vi "Facade.vi"(0 "Data In":T4, 2 "Display State In":T2, 3 "Container State":T3) -> (6 "Data Out":T4, 7 "Display State Out":T2, 8 "Action":T1)   [LabVIEW 2015, in "Scale Selector.xctl"]
uses:
  Scale Selector.xctl
  Data.vi
  <vilib>/_xctls/Container State.ctl
  State.vi
  <vilib>/_xctls/Action.ctl
  <vilib>/_xctls/XControlSupport.lvlib
panel:
  in  "Down Button":bool
  in  "Up Button":bool
  in  "Scale":dbl format="%#pV"
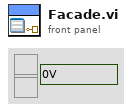
[diagram p1: front panel]
types:
  T1 = typedef "XControlSupport.lvlib/Action.ctl" = cluster{"Data Changed?":bool, "State Changed?":bool, "Action Name":string}
  T2 = typedef "Scale Selector.xctl/State.vi" = cluster{"scale":enum16{"Linear", "Log"}, "increment":dbl}
  T3 = typedef "XControlSupport.lvlib/Container State.ctl" = cluster{"Indicator?":bool, "Run Mode?":bool, " Refnum":refnum<vi>}
  T4 = typedef "Scale Selector.xctl/Data.vi" = dbl
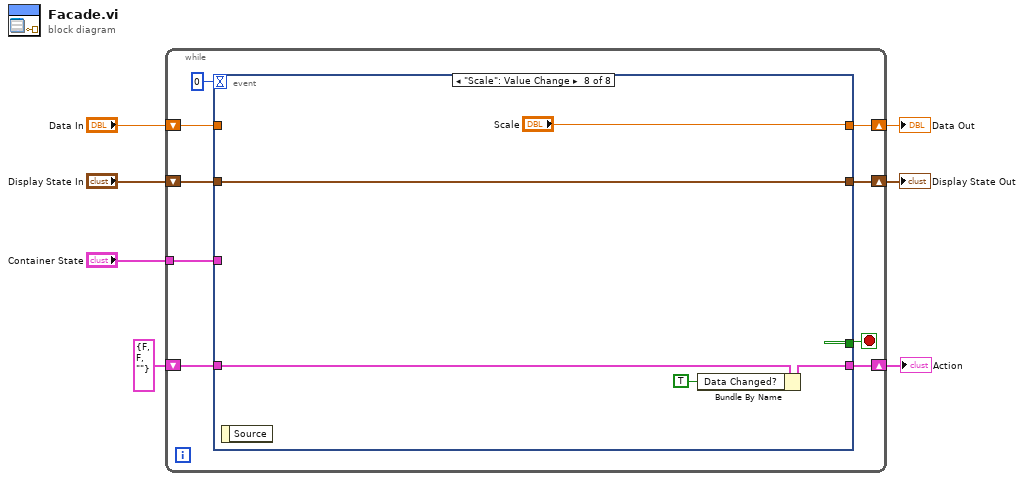
[diagram p0: block diagram]
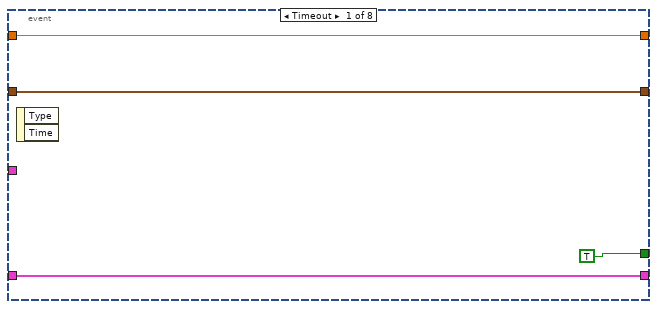
[diagram p2: hidden frame]
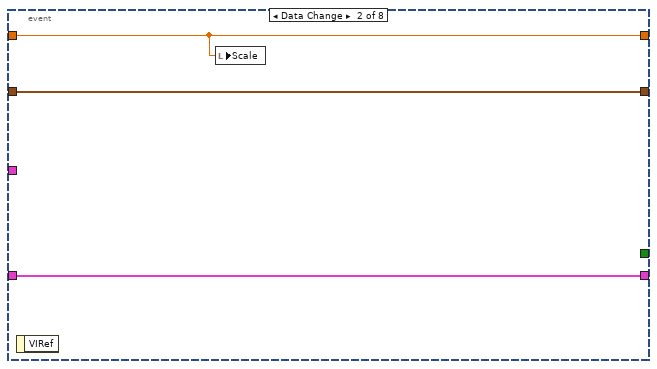
[diagram p3: hidden frame]
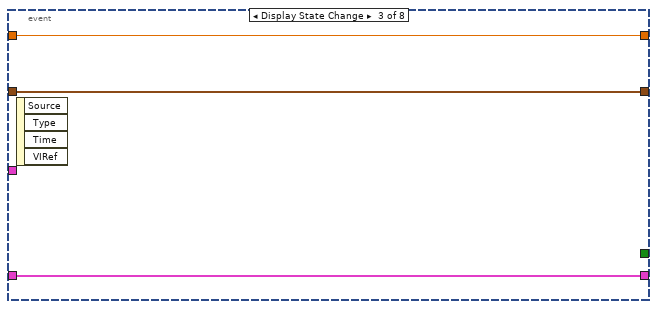
[diagram p4: hidden frame]
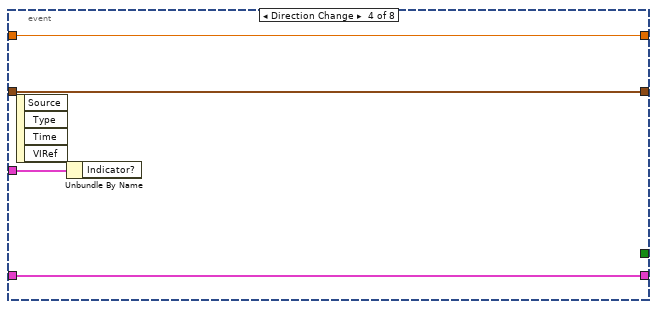
[diagram p5: hidden frame]
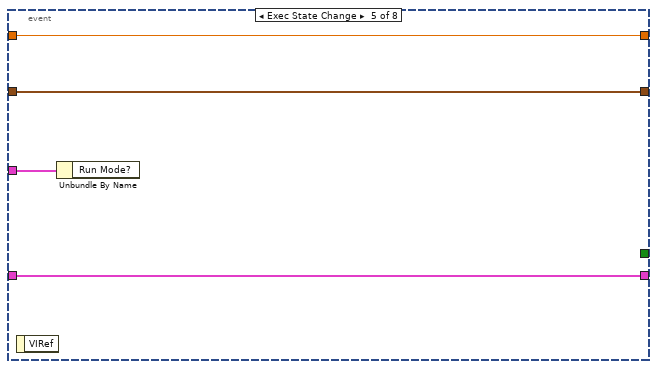
[diagram p6: hidden frame]
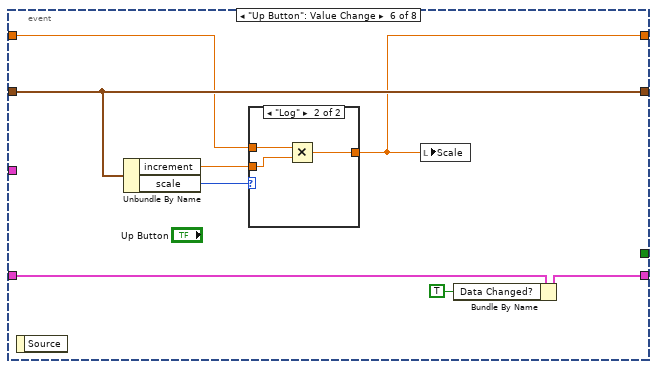
[diagram p7: hidden frame]
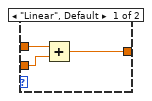
[diagram p8: hidden frame]
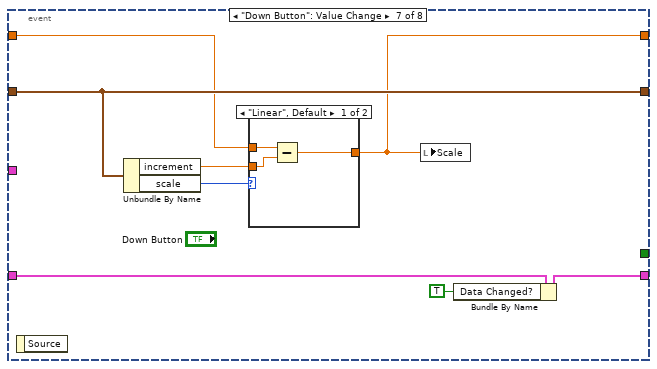
[diagram p9: hidden frame]
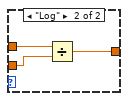
[diagram p10: hidden frame]
diagram:
  n1 = while {
    shift-right: [w15] -> w4
    shift-left: "Display State In" -> [w16]
    tunnel: "Container State" -> [w12]
    shift-right: [w10] -> w7
    shift-left: "Data In" -> [w11]
    shift-right: [w8] -> w2
    shift-left: T1 {"Data Changed?"=FALSE, "State Changed?"=FALSE, "Action Name"=""} ("Action") -> [w9]
    stop <- w14 stop-if-true
    n2 = event shown="[7] \"Scale\": Value Change" {
      selector: _ -> [_ _ _ _ _ _ _ _]
      dyn-events: _ -> [_ _ _ _ _ _ _ _]
      timeout: 0 -> [_ _ _ _ _ _ _ _]
      tunnel: w16 -> [w18 w23 w26 w29 w33 w41 w55 w67]
      tunnel: [w18 w23 w26 w29 w33 w41 w55 w67] -> w15
      tunnel: [TRUE _ _ _ _ _ _ _] -> w14
      tunnel: w12 -> [_ _ _ w30 w34 _ _ _]
      tunnel: w11 -> [w17 w21 w25 w28 w32 w36 w50 _]
      tunnel: [w17 w21 w25 w28 w32 w35 w49 "Scale"] -> w10
      tunnel: [w19 w22 w24 w27 w31 w40 w54 w64] -> w8
      tunnel: w9 -> [w19 w22 w24 w27 w31 w42 w56 w66]
      event Timeout {
        n3 = event-data() -> ()  [unwired: 1 in, 2 out]
      }
      event Data Change {
        n4 = event-data() -> ()  [unwired: 1 in, 1 out]
        n5 = local write "Scale"(w21) -> ()
      }
      event Display State Change {
        n6 = event-data() -> ()  [unwired: 1 in, 4 out]
      }
      event Direction Change {
        n7 = event-data() -> ()  [unwired: 1 in, 4 out]
        n8 = Unbundle By Name(w30) -> ()  [unwired: 1 out]
      }
      event Exec State Change {
        n9 = event-data() -> ()  [unwired: 1 in, 1 out]
        n10 = Unbundle By Name(w34) -> ()  [unwired: 1 out]
      }
      event "Up Button": Value Change {
        n11 = event-data() -> ()  [unwired: 1 in, 1 out]
        n12 = Unbundle By Name(w41) -> ("increment"=w38:dbl, "scale"=w37:enum16{"Linear", "Log"})
        n13 = case shown="\"Log\"" w37 {
          tunnel: w36 -> [w44 w48]
          tunnel: w38 -> [w45 w47]
          tunnel: [w43 w46] -> w35
          frame "Linear", Default {
            n14 = Add(x=w44, y=w45) -> (x+y=w43:T4)
          }
          frame "Log" {
            n15 = Multiply(x=w48, y=w47) -> (x*y=w46:T4)
          }
        }
        n16 = local write "Scale"(w35) -> ()
        n17 = Bundle By Name(cluster=w42, "Data Changed?"=TRUE) -> (w40:T1)
      }
      event "Down Button": Value Change {
        n18 = event-data() -> ()  [unwired: 1 in, 1 out]
        n19 = Unbundle By Name(w55) -> ("increment"=w52:dbl, "scale"=w51:enum16{"Linear", "Log"})
        n20 = case shown="\"Linear\", Default" w51 {
          tunnel: w50 -> [w58 w62]
          tunnel: w52 -> [w59 w61]
          tunnel: [w57 w60] -> w49
          frame "Linear", Default {
            n21 = Subtract(x=w58, y=w59) -> (x-y=w57:T4)
          }
          frame "Log" {
            n22 = Divide(x=w62, y=w61) -> (x/y=w60:T4)
          }
        }
        n23 = local write "Scale"(w49) -> ()
        n24 = Bundle By Name(cluster=w56, "Data Changed?"=TRUE) -> (w54:T1)
      }
      event "Scale": Value Change {
        n25 = event-data() -> ()  [unwired: 1 in, 1 out]
        n26 = Bundle By Name(cluster=w66, "Data Changed?"=TRUE) -> (w64:T1)
      }
    }
  }
  "Display State Out" <- w4
  "Data Out" <- w7
  "Action" <- w2
